vi "Calc Saturated Ampl Multi.vi"(11 "Data":dbl[](array[numeric])) -> (0 "Error":bool, 1 "Errors":dbl[](array[numeric]), 2 "mean":dbl, 3 "Waveform Graph":dbl[][](graph), 4 "Currents":dbl[](array[numeric]))   [LabVIEW 2017]
uses:
  <vilib>/Analysis/baseanly.llb/Mean (DBL).vi
  <vilib>/Analysis/NI_AALBase.lvlib
panel:
  out "Time":u32
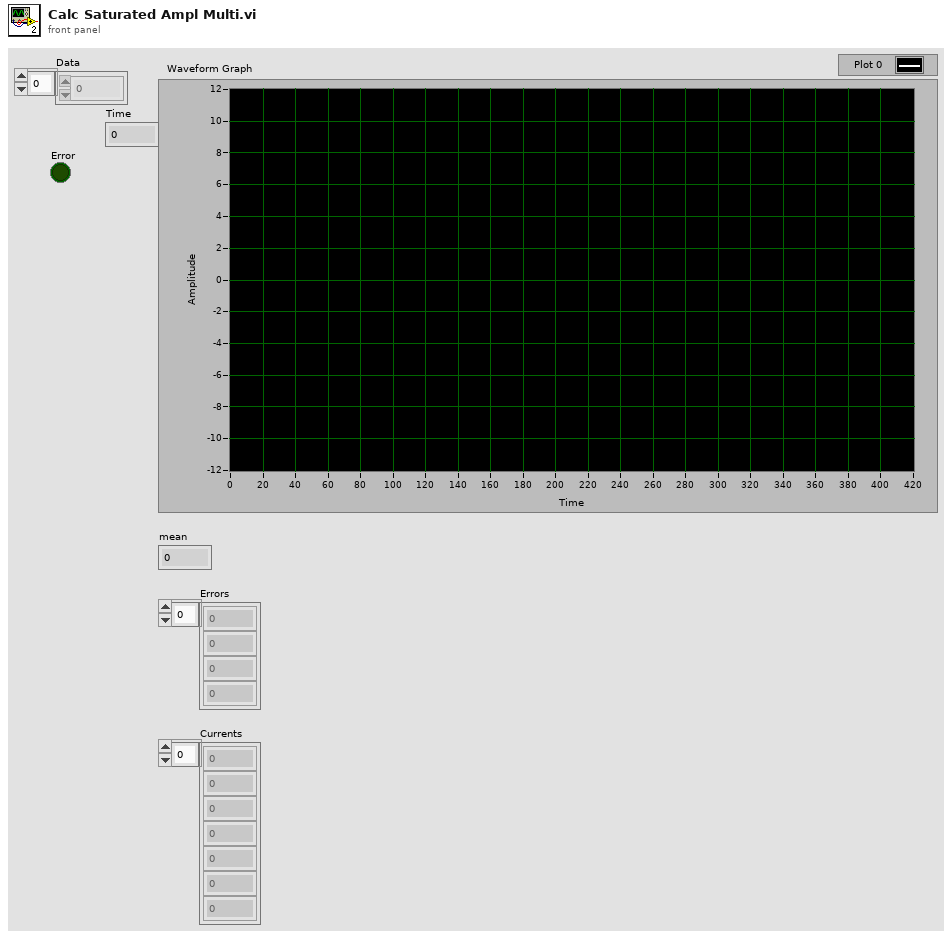
[diagram p1: front panel]
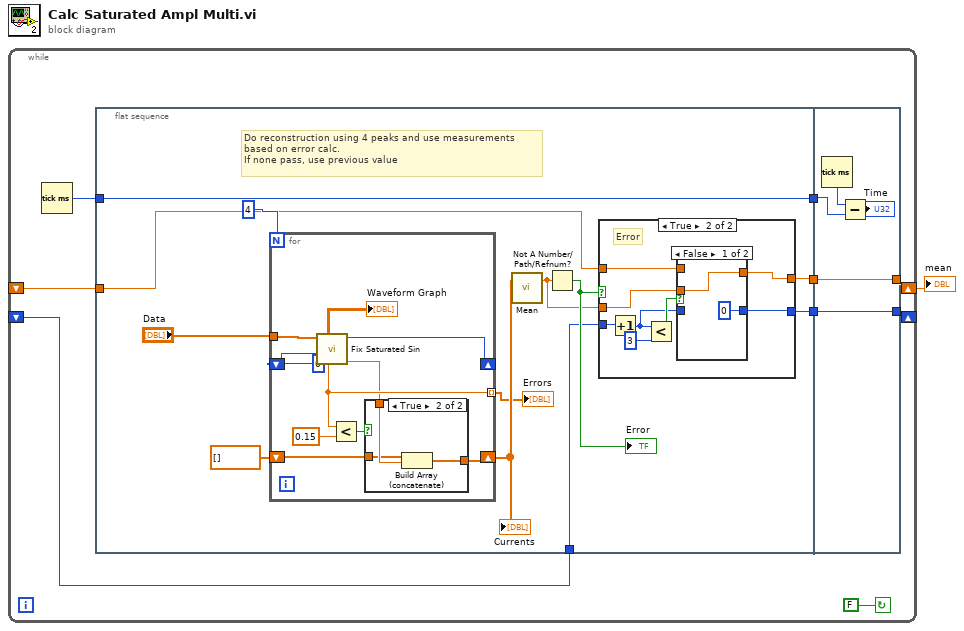
[diagram p0: block diagram]
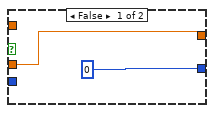
[diagram p2: hidden frame]
diagram:
  n1 = while {
    shift-right: [w5] -> w1
    shift-left: _ -> [w7]
    shift-right: [w4] -> _
    shift-left: _ -> [w2]
    stop <- FALSE continue-if-true
    n2 = Tick Count (ms)() -> (millisecond timer value=w9:u32)
    n3 = flat-sequence {
      tunnel: [w17] -> w10
      tunnel: w9 -> [w17]
      tunnel: w7 -> [w11]
      tunnel: [w13] -> w6
      tunnel: [w15] -> w3
      tunnel: w2 -> [w14]
      tunnel: w10 -> [w55]
      tunnel: [w53] -> w5
      tunnel: w6 -> [w53]
      tunnel: [w52] -> w4
      tunnel: w3 -> [w52]
      frame #0 {
        # "Do reconstruction using 4 peaks and use measurements \nbased on error calc. \nIf none pass, use previous value"
        n4 = for {
          N: 4 -> [_]
          tunnel: "Data" -> [w47]
          shift-right: [w46] -> _
          shift-left: 0 ("Falling") -> [w45]
          tunnel: [w44] -> w21 mode=indexing
          shift-right: [w39] -> w23
          shift-left: dbl[] [] -> [w40]
          n5 = call "Fix Saturated Sin.vi"("start index (0)"=w45, "Waveform"=w47) -> ("RMS value"=w41:dbl, "Falling"=w46:i32, "Error"=w44:dbl, "Waveform Graph"=→"Waveform Graph":dbl[][])  [unwired: 2 in, 4 out]
          n6 = Less?(x=w44, y=0.15) -> (x < y?=w42:bool)
          n7 = case shown="True" w42 {
            tunnel: w41 -> [_ w51]
            tunnel: w40 -> [w48 w50]
            tunnel: [w48 w49] -> w39
            frame False {
            }
            frame True {
              n8 = Build Array (concatenate)(w50, w51) -> (w49:dbl[])
            }
          }
        }
        "Errors" <- w21
        "Currents" <- w23
        n9 = call-poly <vilib>:"Mean.vi"("X"=w23) -> ("mean"=w12:dbl)  [unwired: 1 out]
        n10 = Not A Number/Path/Refnum?(number/path/refnum=w12) -> (NaN/Path/Refnum?=w16:bool)
        "Error" <- w16
        n11 = case shown="True" w16 {
          tunnel: [0 w26] -> w15
          tunnel: w14 -> [_ w33]
          tunnel: [w24 w30] -> w13
          tunnel: w12 -> [w24 w29]
          tunnel: w11 -> [_ w28]
          frame False {
          }
          frame True {
            # "Error"
            n12 = Increment(x=w33) -> (x+1=w27:i32)
            n13 = Less?(x=w27, y=3) -> (x < y?=w31:bool)
            n14 = case shown="False" w31 {
              tunnel: [w35 w37] -> w30
              tunnel: w29 -> [w35 _]
              tunnel: w28 -> [_ w37]
              tunnel: w27 -> [_ w36]
              tunnel: [0 w36] -> w26
              frame False {
              }
              frame True {
              }
            }
          }
        }
      }
      frame #1 {
        n15 = Tick Count (ms)() -> (millisecond timer value=w56:u32)
        n16 = Subtract(x=w56, y=w55) -> (x-y=→"Time":u32)
      }
    }
  }
  "mean" <- w1
